vi "Log Save.vi"(8 "error in (no error)":errorcluster, 10 "Log Msg Line":string, 11 "Log Message":T1) -> (0 "error out":errorcluster, 2 "Complete Log Out":string, 3 "Log Message Out":T1)   [LabVIEW 2026, in "PXI_Common.lvlib"]
uses:
  PXI_Common.lvlib
  Types/Typedef/Log Message.ctl
  Types/Typedef/Log Message Levels.ctl
  Types/Enum/Bench Modules.ctl
  Paths/Items/Temp Path.vi
  <vilib>/Utility/Data Type/NI_Data Type.lvlib
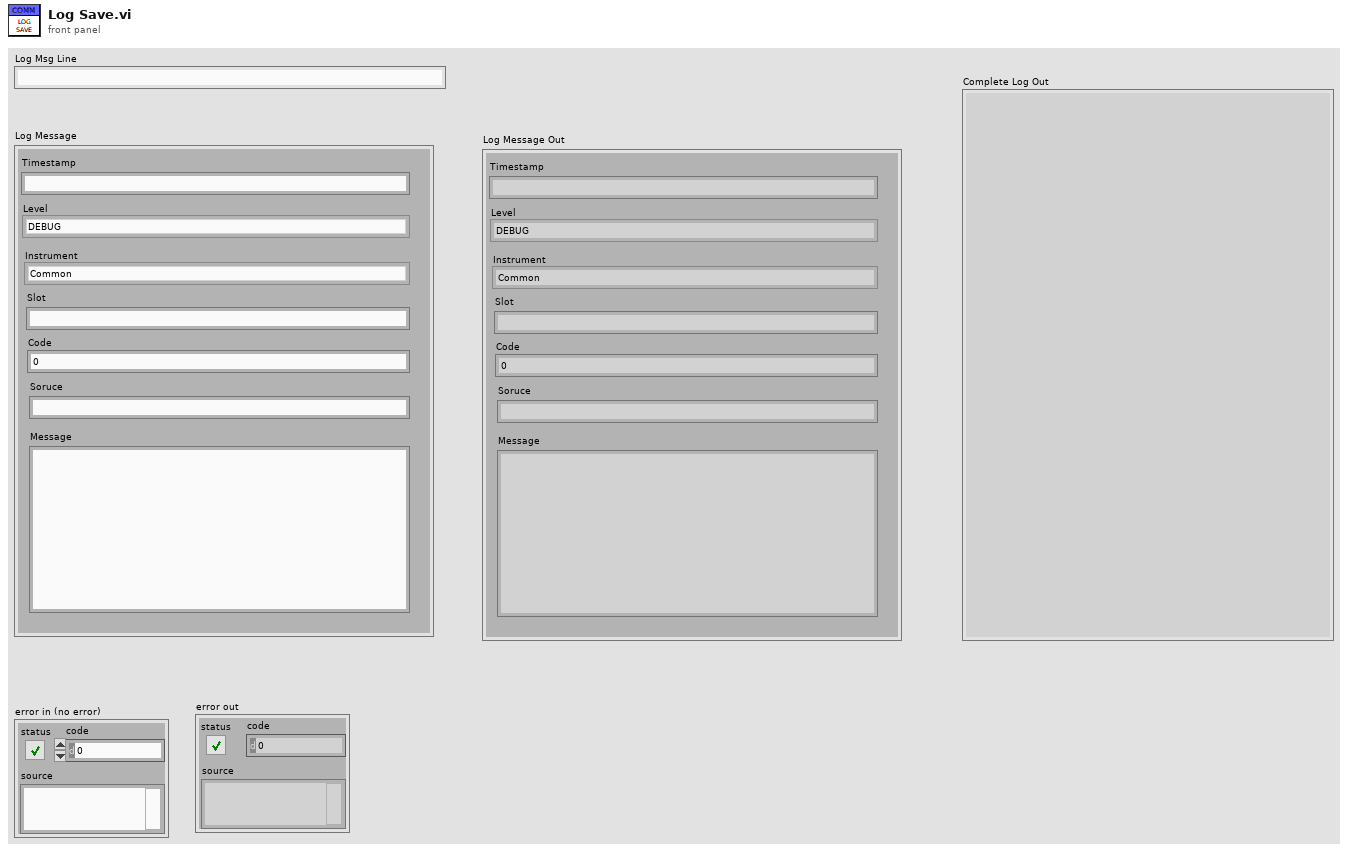
[diagram p1: front panel]
types:
  T1 = typedef "PXI_Common.lvlib/Log Message.ctl" = cluster{"Timestamp":string, "Level":T2, "Instrument":T3, "Slot":string, "Code":i32, "Soruce":string, "Message":string}
  T2 = typedef "PXI_Common.lvlib/Log Message Levels.ctl" = enum16{"DEBUG", "INFO", "WARNING", "ERROR"}
  T3 = typedef "PXI_Common.lvlib/Bench Modules.ctl" = enum16{"Common", "PXI4072", "PXI6259", "PXI6224", "PXI4130", "PXI8431"}
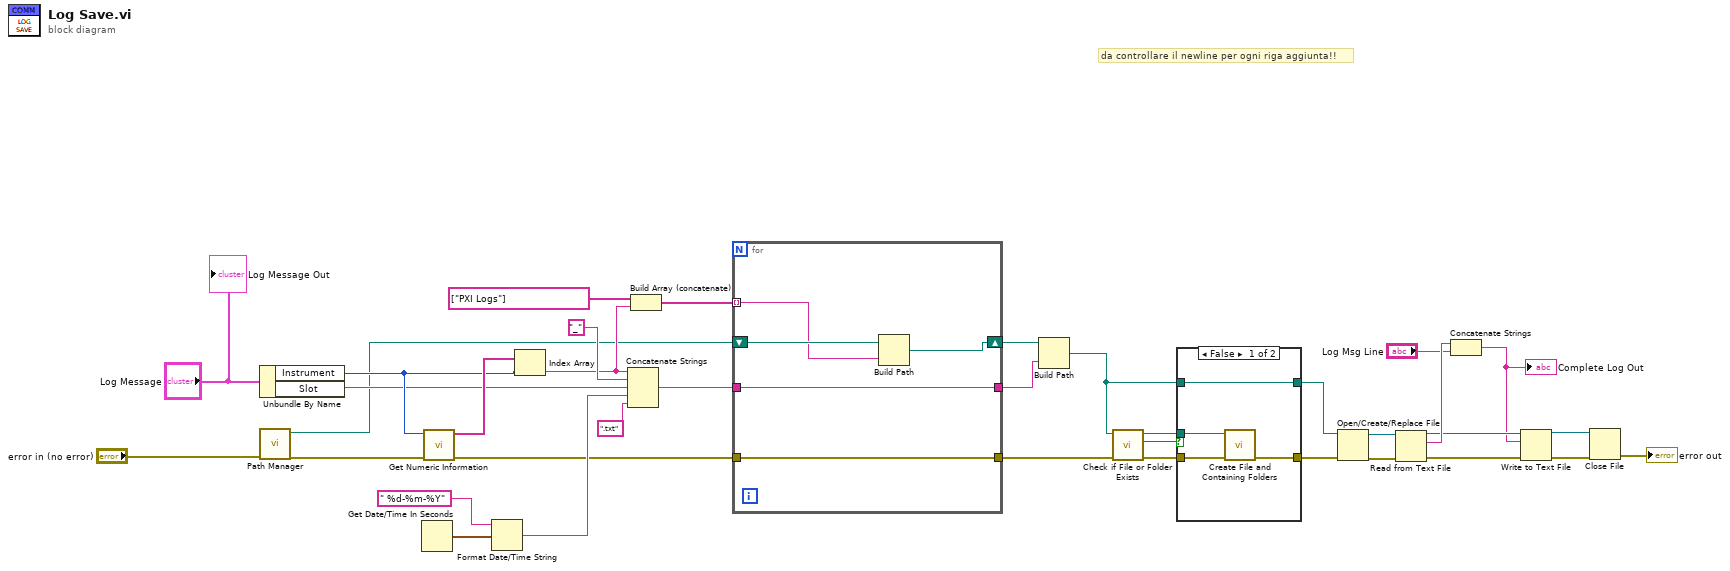
[diagram p0: block diagram]
diagram:
  # "da controllare il newline per ogni riga aggiunta!!"
  n1 = Unbundle By Name("Log Message") -> ("Instrument"=w32:T3, "Slot"=w30:string)
  n2 = call-poly "Path Manager.vi"("error in (no error)"="error in (no error)") -> ("error out"=w34:errorcluster, "path"=w22:path)  [unwired: 9 in]
  n3 = Get Date/Time In Seconds() -> (seconds since 1Jan1904=w29:timestamp)
  n4 = call <vilib>:"Get Numeric Information.vi"("error in (no error)"=w34, "variant"=w32) -> ("error out"=w21:errorcluster, "enum names"=w33:string[])  [unwired: 6 in, 2 out]
  n5 = Format Date/Time String(time format string (%c)=" %d-%m-%Y", seconds (now)=w29) -> (date/time string=w27:string)  [unwired: 1 in]
  n6 = Index Array(array=w33, index=w32) -> (element=w24:string)
  n7 = Concatenate Strings(w24, "_", w30, w27, ".txt" ("string")) -> (w20:string)
  n8 = Build Array (concatenate)(string[] ["PXI Logs"], w24) -> (w23:string[])
  n9 = for {
    tunnel: w23 -> [w40] mode=indexing
    tunnel: w21 -> [w37]
    shift-right: [w39] -> w19
    shift-left: w22 -> [w41]
    tunnel: w20 -> [w38]
    tunnel: [w38] -> w18
    tunnel: [w37] -> w17
    n10 = Build Path(base path=w41, name or relative path=w40) -> (appended path=w39:path)
  }
  n11 = Build Path(base path=w19, name or relative path=w18) -> (appended path=w12:path)
  n12 = call <vilib>:"Check if File or Folder Exists.vi"("error in (no error)"=w17, "path"=w12) -> ("error out"=w15:errorcluster, "file or folder exists?"=w16:bool, "dup path"=w14:path)  [unwired: 7 in]
  n13 = case shown="False" w16 {
    tunnel: w15 -> [w45 w46]
    tunnel: w14 -> [w44 _]
    tunnel: [w43 w46] -> w13
    tunnel: w12 -> [w42 w47]
    tunnel: [w42 w47] -> w11
    frame False {
      n14 = call <vilib>:"Create File and Containing Folders.vi"("error in (no error)"=w45, "file path"=w44) -> ("error out"=w43:errorcluster)  [unwired: 8 in, 1 out]
    }
    frame True {
    }
  }
  n15 = Open/Create/Replace File(file path (use dialog)=w11, error in=w13) -> (refnum out=w6:refnum<file>, error out=w7:errorcluster)  [unwired: 4 in, 1 out]
  n16 = Read from Text File(file (use dialog)=w6, error in=w7) -> (refnum out=w3:refnum<file>, text=w5:string, error out=w1:errorcluster)  [unwired: 2 in, 1 out]
  n17 = Concatenate Strings(w5, "Log Msg Line") -> (w2:string)
  "Complete Log Out" <- w2
  n18 = Write to Text File(file (use dialog)=w3, text=w2, error in=w1) -> (refnum out=w8:refnum<file>, error out=w10:errorcluster)  [unwired: 1 in, 1 out]
  n19 = Close File(refnum=w8, error in=w10) -> (error out=→"error out":errorcluster)  [unwired: 1 out]
  "Log Message Out" <- "Log Message"
